vi "getDescription.vi"(8 "error in (no error)":errorcluster, 11 "HouseBlend in":refnum<class "HouseBlend.lvclass">) -> (0 "error out":errorcluster, 2 "description":string, 3 "HouseBlend out":refnum<class "HouseBlend.lvclass">)   [LabVIEW 2017, in "HouseBlend.lvclass"]
uses:
  HouseBlend.lvclass
  Beverage Class/Beverage.lvclass
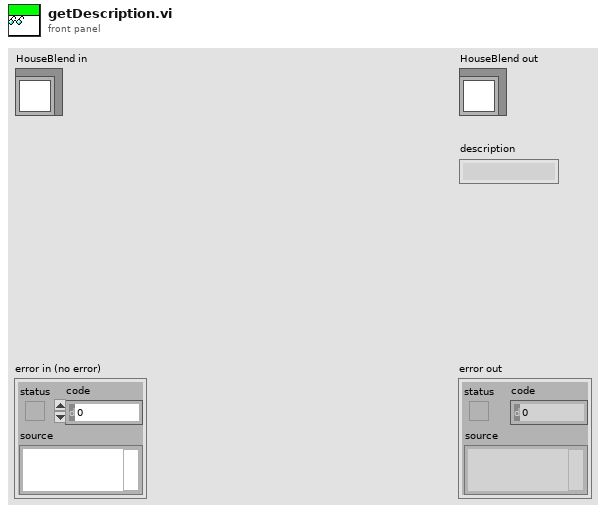
[diagram p1: front panel]
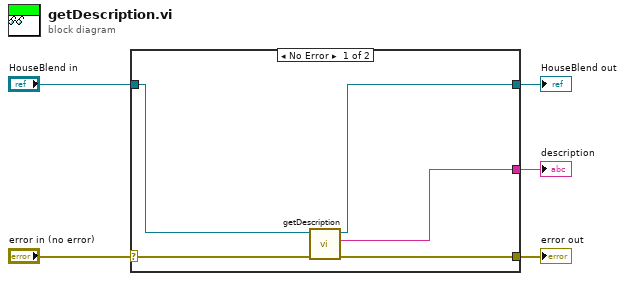
[diagram p0: block diagram]
diagram:
  n1 = case shown="No Error" "error in (no error)" {
    selector: "error in (no error)" -> [w10 w11]
    tunnel: [w9 w11] -> w4
    tunnel: [w7 w12] -> w2
    tunnel: "HouseBlend in" -> [w8 w12]
    tunnel: [w6 _] -> w1
    frame No Error {
      n2 = call-parent "getDescription.vi"("error in (no error)"=w10, "Beverage in"=w8) -> ("error out"=w9:errorcluster, "description"=w6:string, "Beverage out"=w7:refnum<class "HouseBlend.lvclass">)  [unwired: 7 in]
    }
    frame Error {
    }
  }
  "error out" <- w4
  "HouseBlend out" <- w2
  "description" <- w1
